vi "Eyes.vi"() -> ()   [LabVIEW 2020]
uses:
  <vilib>/measure/matone.llb/Extract Single Tone Information 1 Chan.vi
  <vilib>/express/express analysis/Spectral/Block/exnSpectralBlock spectral measurements peak poly.vi
  <vilib>/express/express analysis/Spectral/Block/exnSpectralBlock spectral measurements peak WFM.vi
  <vilib>/Analysis/1siggen.llb/Ramp Pattern by Delta.vi
  <vilib>/express/express analysis/Spectral/XNode/ExpressSpectralMeasurementsBlockNode.xnode
  <vilib>/DigilentWF/DigilentWF.lvlib
  <vilib>/Analysis/NI_AALBase.lvlib
  <vilib>/measure/NI_MAPro.lvlib
panel:
  in  "Threshold":dbl=2.0
  out "Eyes Closed?":bool
  out "Peak Frequency\nAbout 8 to 12 Hz":dbl
  in  "Max Fequency":dbl=80.0
  out "FFT":cluster{"Ramp Pattern":dbl[], "magnitude":dbl[]}(graph)
  out "Signal":waveform(dbl)(graph)
  out "error out":errorcluster
  in  "?":bool
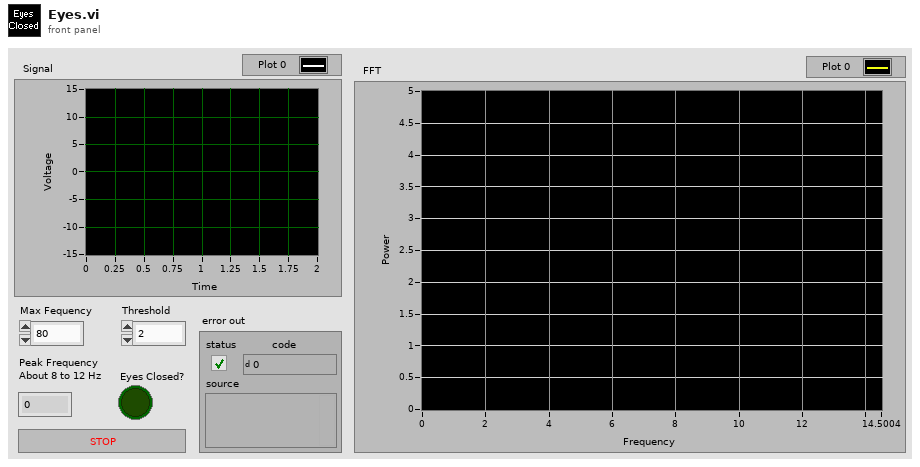
[diagram p1: front panel]
types:
  T1 = enum32{"none", "input signal", "detected signal", "residual signal"}
  T2 = cluster{"averaging mode":u16, "weighting mode":u16, "number of averages":u32}
  T3 = cluster{"dB On (F)":bool, "unwrap phase (F)":bool, "convert to degree (F)":bool}
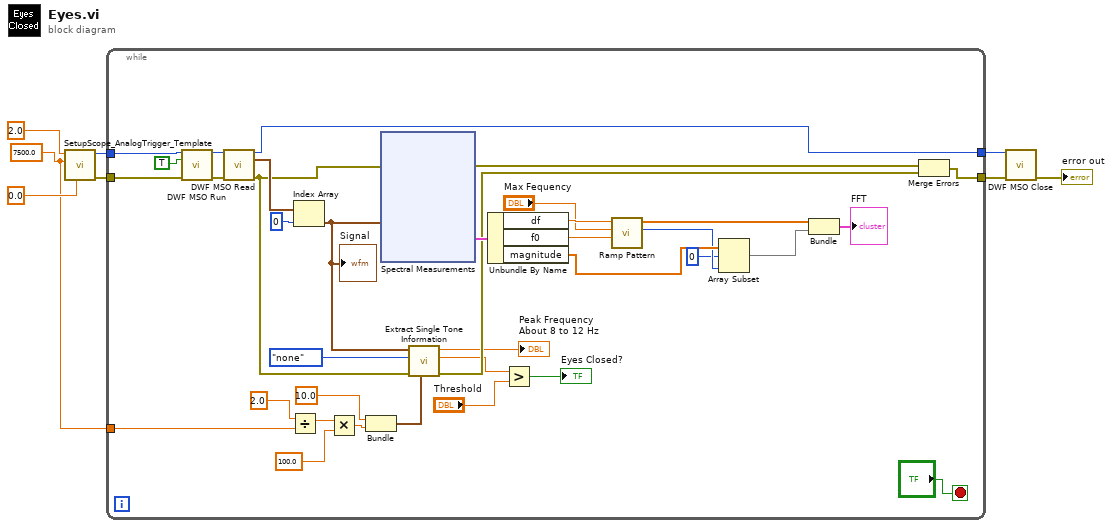
[diagram p0: block diagram]
diagram:
  w1 = 7500.0
  n1 = call "SetupScope_AnalogTrigger_Template.vi"("Trigger Level"=0.0, "Sample Rate (Hz)"=w1, "Acquisition\nTime Length (s)"=2.0) -> ("error out"=w7:errorcluster, "MSO Instrument Handle Out"=w6:u32)  [unwired: 7 in]
  n2 = while {
    tunnel: w7 -> [w43]
    tunnel: w6 -> [w42]
    tunnel: [w27] -> w4
    tunnel: [w38] -> w3
    tunnel: w1 -> [w15]
    stop <- "?" stop-if-true
    n3 = call <vilib>:"DWF MSO Run.vi"("Instrument Handle In"=w42, "Auto Trigger"=TRUE, "Error In"=w43) -> ("Instrument Handle Out"=w41:u32, "Error Out"=w40:errorcluster)  [unwired: 11 in]
    n4 = call <vilib>:"DWF MSO Read.vi"("Instrument Handle In"=w41, "Error In"=w40) -> ("Instrument Handle Out"=w38:u32, "Analog Waveforms"=w36:waveform(dbl)[], "Error Out"=w21:errorcluster)  [unwired: 8 in, 3 out]
    n5 = Divide(x=2.0, y=w15) -> (x/y=w18:dbl)
    n6 = Index Array "Index Array"(array=w36, index=0) -> (element=w23:waveform(dbl))
    "Signal" <- w23
    n7 = Multiply(x=w18, y=100.0) -> (x*y=w19:dbl)
    n8 = Bundle(10.0, w19) -> (w17:cluster{dbl, dbl})  [unwired: 1 in]
    n9 = xnode "Spectral Measurements"("Signals"=w23, "error in (no error)"=w21) -> ("FFT - (Peak)"=w35:cluster{"f0":dbl, "df":dbl, "magnitude":dbl[]}, "error out"=w26:errorcluster)  [unwired: 1 out]
    n10 = call-poly <vilib>:"Extract Single Tone Information.vi"("advanced search"=w17, "error in (no error)"=w21, "export mode"=T1."none", "time signal in"=w23) -> ("error out"=w14:errorcluster, "detected amplitude"=w9:dbl, "detected frequency"=→"Peak Frequency\nAbout 8 to 12 Hz":dbl)  [unwired: 2 in, 3 out]
    n11 = Unbundle By Name(w35) -> ("df"=w33:dbl, "f0"=w34:dbl, "magnitude"=w31:dbl[])
    n12 = Greater?(x=w9, y="Threshold") -> (0:→"Eyes Closed?":bool)
    n13 = call-poly <vilib>:"Ramp Pattern.vi"("start"=w34, "end"="Max Fequency", "delta"=w33) -> ("samples"=w30:i32, "Ramp Pattern"=w24:dbl[])  [unwired: 6 in, 1 out]
    n14 = Array Subset "Array Subset"(array=w31, index=0, length=w30) -> (w25:dbl[])
    n15 = Bundle("Ramp Pattern"=w24, w25) -> (→"FFT":cluster{"Ramp Pattern":dbl[], dbl[]})  [unwired: 1 in]
    n16 = Merge Errors(w26, w14) -> (w27:errorcluster)
  }
  n17 = call <vilib>:"DWF MSO Close.vi"("Instrument Handle In"=w3, "Error In"=w4) -> ("Error Out"=→"error out":errorcluster)  [unwired: 13 in]
